vi "LimitStringWidthInPixels.vi"(0 "String":string, 5 "Max string width":i16 caption="Max string width [pixels]", 7 "Append ellipsis?":bool=TRUE caption="Append ellipsis? (T)", 9 "Desired font":T2(ring)=enum."Application Font" caption="Desired font (Application)", 11 "User-specified font":T1) -> (4 "Final string":string, 6 "Final string width":i16 caption="Final string width [pixels]", 8 "Target width achieved?":bool, 10 "String modified?":bool)   [LabVIEW 2017, in "GPString.lvlib"]
doc: "Reduces <B>String</B> in length until it fits within <B>Max string width</B> in pixels.\n\nThis function creates a graphic of the string to calculate its resulting width in pixels, using <B>Desired font</B> and optionally the <B>User-specified font</B> setting if <B>Desired font</B> is set to 'User-specified Font'.\n\nThe optional <B>Append ellipsis?</B> lets you select if the string should have an ellipsis (...) appended in case the string gets truncated to fit the target width.\n\nThe truncation attempt stops when <B>Final string</B> reaches a single character (plus the optional ellipsis), in which case <B>Target width achieved?</B> could still be False.\n\nThis VI is inlined.\n\nSteen Schmidt\nGPower\n12/11 2013"
uses:
  GPString.lvlib
panel:
  # "Copyright © 2016\nGPower\nSee enclosed license file for terms and conditions"
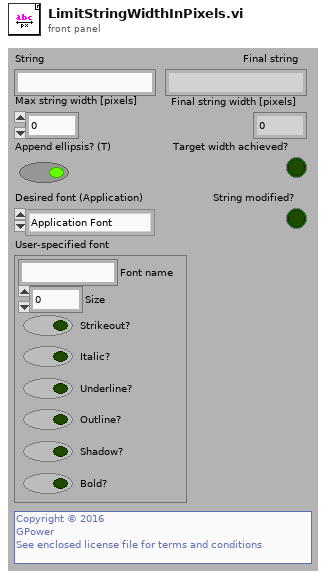
[diagram p1: front panel]
types:
  T1 = cluster{"Font name":string, "Size":i16, "Strikeout?":bool, "Italic?":bool, "Underline?":bool, "Outline?":bool, "Shadow?":bool, "Bold?":bool}
  T2 = enum16{"User-specified Font", "Application Font", "System Font", "Dialog Font"}
  T3 = cluster{"left":i16, "top":i16, "right":i16, "bottom":i16}
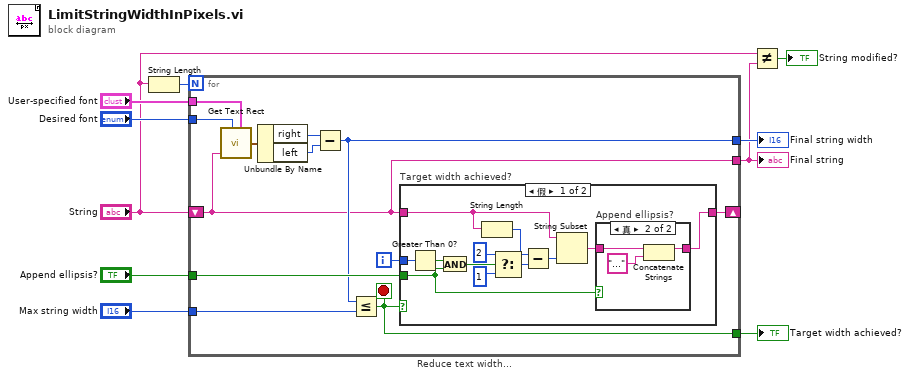
[diagram p0: block diagram]
diagram:
  n1 = String Length(string="String") -> (length=w4:i32)
  n2 = for "Reduce text width..." {
    N: w4 -> [_]
    tunnel: "Desired font" -> [w21]
    tunnel: "User-specified font" -> [w20]
    shift-right: [w16] -> _
    shift-left: "String" -> [w12]
    tunnel: "Max string width" -> [w17]
    tunnel: "Append ellipsis?" -> [w14]
    tunnel: [w13] -> w6
    tunnel: [w12] -> w3
    tunnel: [w11] -> w5
    i -> [w15]
    stop <- w11 stop-if-true
    n3 = call <vilib>:"Get Text Rect.vi"("desired font(Application)"=w21, "text"=w12, "[user-specified font]"=w20) -> ("rect"=w22:T3)  [unwired: 6 in]
    n4 = Unbundle By Name(w22) -> ("right"=w19:i16, "left"=w18:i16)
    n5 = Subtract(x=w19, y=w18) -> (x-y=w13:i16)
    n6 = Less Or Equal?(x=w13, y=w17) -> (x <= y?=w11:bool)
    n7 = case "Target width achieved?" shown="假" w11 {
      tunnel: w12 -> [w26 w39]
      tunnel: [w27 w39] -> w16
      tunnel: w15 -> [w34 _]
      tunnel: w14 -> [w29 _]
      frame False {
        n8 = Greater Than 0?(x=w34) -> (x > 0?=w33:bool)
        n9 = And(x=w33, y=w29) -> (x .and. y?=w32:bool)
        n10 = String Length(string=w26) -> (length=w25:i32)
        n11 = Select(t=2, s=w32, f=1) -> (s? t:f=w24:i32)
        n12 = Subtract(x=w25, y=w24) -> (x-y=w23:i32)
        n13 = String Subset(string=w26, length (rest)=w23) -> (substring=w28:string)  [unwired: 1 in]
        n14 = case "Append ellipsis?" shown="真" w29 {
          tunnel: w28 -> [w35 w37]
          tunnel: [w35 w36] -> w27
          frame False {
          }
          frame True {
            n15 = Concatenate Strings(w37, "…") -> (w36:string)
          }
        }
      }
      frame True {
      }
    }
  }
  "Final string" <- w3
  "Target width achieved?" <- w5
  "Final string width" <- w6
  n16 = Not Equal?(x="String", y=w3) -> (x != y?=→"String modified?":bool)
